vi "citire salvare date.vi"(8 "NN- Trained file name":path, 11 "Dataset folder":path) -> (0 "RN outputs":i32, 1 "DataSet Trainded data":path, 2 "Inputs":i32, 3 "DataSet File":path[][](array[path]), 4 "nume clase":string[](array[string]))   [LabVIEW 2024]
uses:
  <vilib>/National Instruments/NI Super Simple Neural Networks/Types/Teaching Vector.ctl
  <vilib>/National Instruments/NI Super Simple Neural Networks/Types/1D Array.ctl
  <vilib>/National Instruments/NI Super Simple Neural Networks/Neural Network.lvclass
panel:
  out "appended path":path
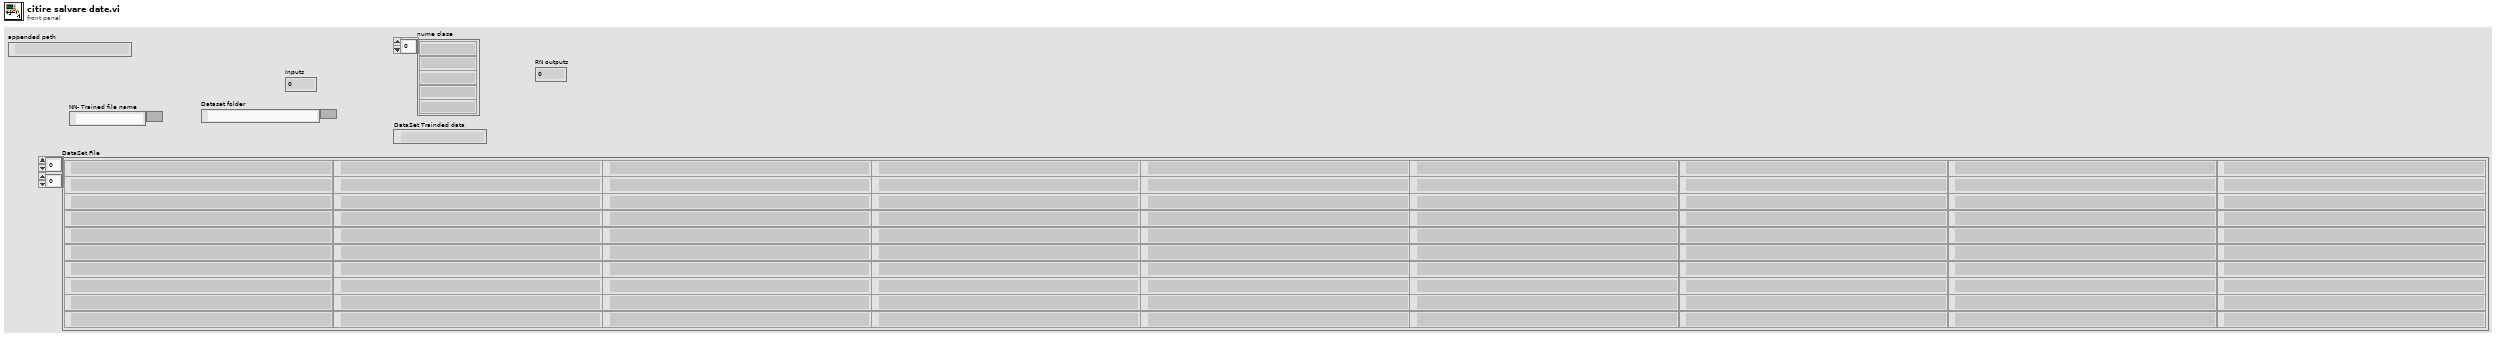
[diagram p1: front panel]
types:
  T1 = enum16{"open", "replace", "create", "open or create", "replace or create", "replace or create with confirmation"}
  T2 = enum16{"Normalizare [0,1]", "Normalizare[-1,1]", "Fara normalizare"}
  T3 = typedef "Neural Network.lvclass/Teaching Vector.ctl" = cluster{"Inputs":T4, "Expected Outputs":T4}
  T4 = typedef "Neural Network.lvclass/1D Array.ctl" = cluster{"1D Array":dbl[]}
  T5 = typedef "imagedata.ctl" = cluster{"image type":i32, "image depth":i32, "image":u8[], "mask":u8[], "colors":u32[], "Rectangle":cluster{"left":i16, "top":i16, "right":i16, "bottom":i16}}
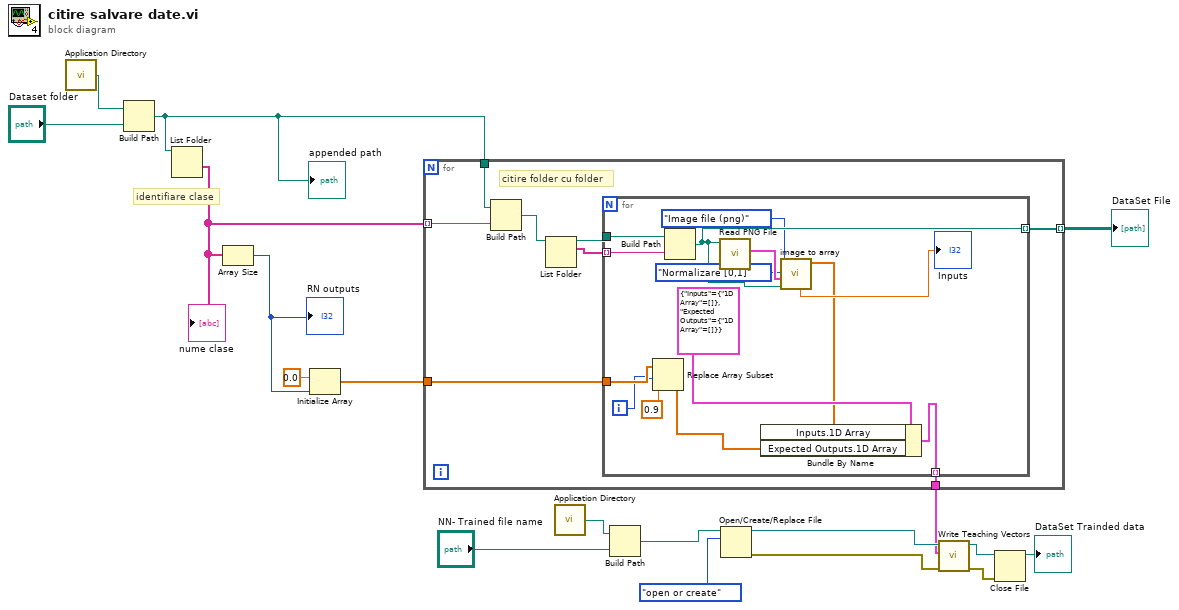
[diagram p0: block diagram]
diagram:
  # "identifiare clase"
  n1 = call <vilib>:"Application Directory.vi"() -> ("Application Directory"=w18:path)
  n2 = Build Path(base path=w18, name or relative path="Dataset folder") -> (appended path=w1:path)
  "appended path" <- w1
  n3 = List Folder(path=w1) -> (folder names=w14:string[])  [unwired: 3 in, 3 out]
  "nume clase" <- w14
  n4 = Array Size(array=w14) -> (size(s)=w16:i32)
  "RN outputs" <- w16
  n5 = Initialize Array(0.0 ("element"), w16) -> (w13:dbl[])
  n6 = for {
    tunnel: w1 -> [w26]
    tunnel: w14 -> [w25] mode=indexing
    tunnel: w13 -> [w23]
    tunnel: [w22] -> w6
    tunnel: [w21] -> w2 mode=indexing
    # "citire folder cu folder"
    n7 = Build Path(base path=w26, name or relative path=w25) -> (appended path=w20:path)
    n8 = List Folder(path=w20) -> (path out=w24:path, filenames=w19:string[])  [unwired: 3 in, 2 out]
    n9 = for {
      tunnel: w24 -> [w40]
      tunnel: w23 -> [w39]
      tunnel: [w35] -> w22 mode=indexing
      tunnel: [w32] -> w21 mode=indexing
      tunnel: w19 -> [w34] mode=indexing
      i -> [w33]
      n10 = Replace Array Subset(array=w39, new element=0.9 ("new element/subarray"), index=w33) -> (w37:dbl[])
      n11 = Build Path(base path=w40, name or relative path=w34) -> (appended path=w32:path)
      n12 = call <vilib>:"Read PNG File.vi"("path to PNG file"=w32) -> ("image data"=w31:T5)  [unwired: 8 in, 2 out]
      n13 = call "image to array.vi"("Path to PNG file"=w32, "image data"=w31, "Normalizare"=T2."Normalizare [0,1]", "Image type"=enum16{"Image file (png)", "Image data"}."Image file (png)") -> ("Image 1d Array"=w29:dbl[], "Nr.pixeli"=→"Inputs":dbl)  [unwired: 3 in, 3 out]
      n14 = Bundle By Name(cluster=T3 {"Inputs"={"1D Array"=[]}, "Expected Outputs"={"1D Array"=[]}} ("Teaching Vector"), "Inputs.1D Array"=w29, "Expected Outputs.1D Array"=w37) -> (w35:T3)
    }
  }
  "DataSet File" <- w2
  n15 = call <vilib>:"Application Directory.vi"() -> ("Application Directory"=w12:path)
  n16 = Build Path(base path=w12, name or relative path="NN- Trained file name") -> (appended path=w10:path)
  n17 = Open/Create/Replace File(file path (use dialog)=w10, operation (0:open)=T1."open or create") -> (refnum out=w7:refnum<file>, error out=w8:errorcluster)  [unwired: 4 in, 1 out]
  n18 = call <vilib>:"Write Teaching Vectors.vi"("Error In"=w8, "Teaching Vectors"=w6, "Teaching File Ref In"=w7) -> ("Error Out"=w4:errorcluster, "Teaching File Ref Out"=w5:refnum<file>)  [unwired: 7 in]
  n19 = Close File(refnum=w5, error in=w4) -> (path=→"DataSet Trainded data":path)  [unwired: 1 out]
